vi "CSM_Item_Init.vi"(11 "Object":T1) -> ()   [LabVIEW 2014]
uses:
  <resource>/Framework/Providers/API/ItemRef.ctl
  <resource>/Framework/Providers/API/mxLvMenuItem.ctl
panel:
  out "error out":errorcluster
  in  "error in":errorcluster
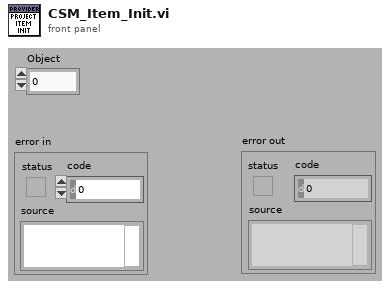
[diagram p1: front panel]
types:
  T1 = typedef "ItemRef.ctl" = u64
  T2 = typedef "mxLvMenuItem.ctl" = cluster{"Menu Name":string, "Description":string, "Icon File Name":path, "Menu Tag":string, "Enabled":bool, "Checked":bool, "Separator":bool, "Batchable":bool, "Weight":i32, "Batch Mode (Ignored if Not Batchable)":enum32{"Show If All Items Support Command", "Show If Any Items Support Command"}, "Menu Location":enum32{"<None>", "Project", "Project / Build Specifications", "Tools", "Tools / Source Control", "Tools / Real-Time Module", "Help"}, "Exclude From Getting Started Window Menu":bool}
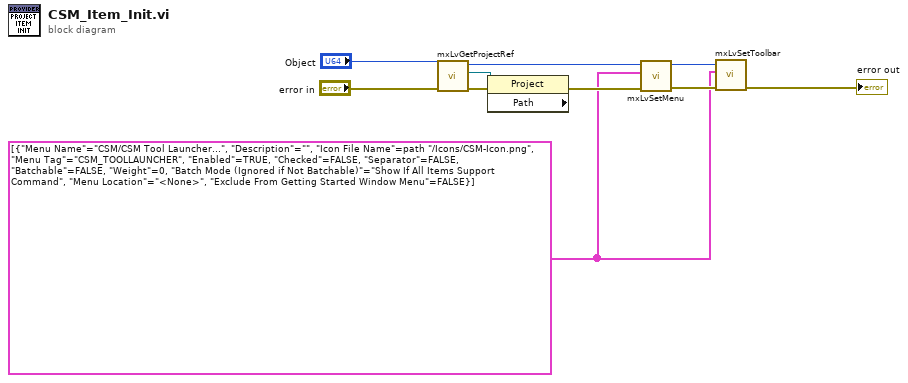
[diagram p0: block diagram]
diagram:
  w1 = T2[] [{"Menu Name"="CSM/CSM Tool Launcher...", "Description"="", "Icon File Name"=path "../Icons/CSM-Icon.png", "Menu Tag"="CSM_TOOLLAUNCHER", "Enabled"=TRUE, "Checked"=FALSE, "Separator"=FALSE, "Batchable"=FALSE, "Weight"=0, "Batch Mode (Ignored if Not Batchable)"=enum."Show If All Items Support Command", "Menu Location"=enum."<None>", "Exclude From Getting Started Window Menu"=FALSE}] ("Array in")
  n1 = call <resource>:"mxLvGetProjectRef.vi"("error in"="error in", "Item"="Object") -> ("error out"=w8:errorcluster, "Project Refnum"=w7:refnum<vi>, "Item"=w6:T1)  [unwired: 7 in]
  n2 = property class="Project" props=["Path"](reference=w7, error in=w8) -> (error out=w5:errorcluster)  [unwired: 2 out]
  n3 = call <resource>:"mxLvSetMenu.vi"("error in"=w5, "Menu Items"=w1, "Item"=w6) -> ("error out"=w9:errorcluster, "Item"=w10:T1)  [unwired: 7 out]
  n4 = call <resource>:"mxLvSetToolbar.vi"("error in"=w9, "Toolbar Items"=w1, "Item"=w10) -> ("error out"=→"error out":errorcluster)  [unwired: 7 in, 1 out]
